vi "arm during load cancel.vi"(1 "Arm Canceled During Load?":bool, 2 "Mode":enum16{"Get", "Set", "Teleop Set"}(ring)) -> (0 "Arm Canceled During Load":bool)   [LabVIEW 2013]
panel:
  # "A FG To Allow Arm to be Canceled During Load Without a Major Catastrophic Failure"
  # "(not really, but it would be a major setback during a match without this)"
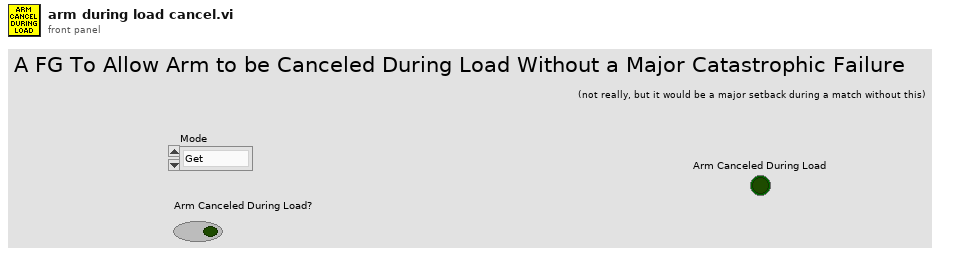
[diagram p1: front panel]
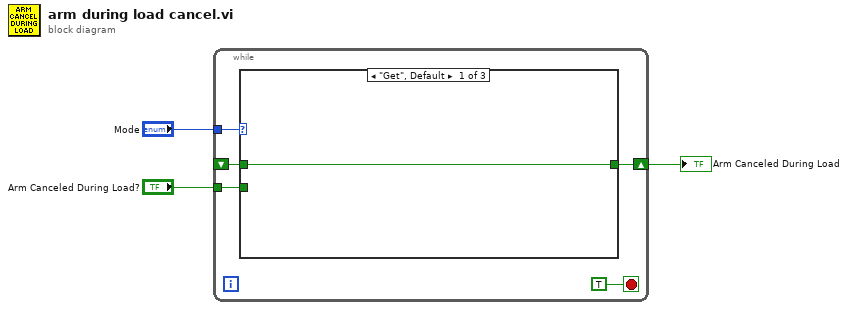
[diagram p0: block diagram]
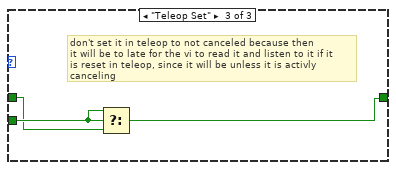
[diagram p3: hidden frame]
diagram:
  n1 = while {
    tunnel: "Mode" -> [w7]
    tunnel: "Arm Canceled During Load?" -> [w6]
    shift-right: [w5] -> w2
    shift-left: _ -> [w4]
    stop <- TRUE stop-if-true
    n2 = case shown="\"Get\", Default" w7 {
      tunnel: w6 -> [_ w10 w13]
      tunnel: [w9 w10 w11] -> w5
      tunnel: w4 -> [w9 _ w12]
      frame "Get", Default {
      }
      frame "Set" {
      }
      frame "Teleop Set" {
        # "don't set it in teleop to not canceled because then\nit will be to late for the vi to read it and listen to it if it\nis reset in teleop, since it will be unless it is activly canceling"
        n3 = Select(t=w13, s=w13, f=w12) -> (s? t:f=w11:bool)
      }
    }
  }
  "Arm Canceled During Load" <- w2
